vi "Unescape Type Name.vi"(10 "String":string) -> (2 "String out":string)   [LabVIEW 2017, in "Flatten To JSON Object.lvclass"]
doc: "Unescapes the type name from a JSON text value."
uses:
  Flatten To JSON Object.lvclass
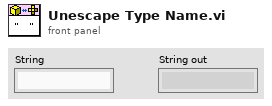
[diagram p1: front panel]
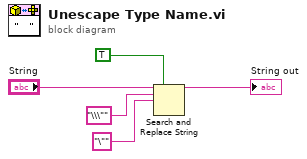
[diagram p0: block diagram]
diagram:
  n1 = Search and Replace String(replace all?=TRUE ("replace all? (F)"), input string="String", search string="\\\"" ("input string"), replace string="\"" ("search string")) -> (result string=→"String out":string)  [unwired: 4 in, 3 out]
